vi "IsStringConstant__slk_mt.vi"(7 "create enum configure":T1, 8 "error in (no error)":errorcluster, 11 "selection list":refnum<vi>[](array[refnum])) -> (0 "error out":errorcluster, 2 "position":cluster{"Left":i32, "Top":i32}, 3 "values":string[](array[string]), 4 "not?":bool)   [LabVIEW 2010]
uses:
  TypeDef/TypeDef_CreateEnumConfigure__slk_mt.ctl
  Library/Lazyboots Menu Tool.lvlib
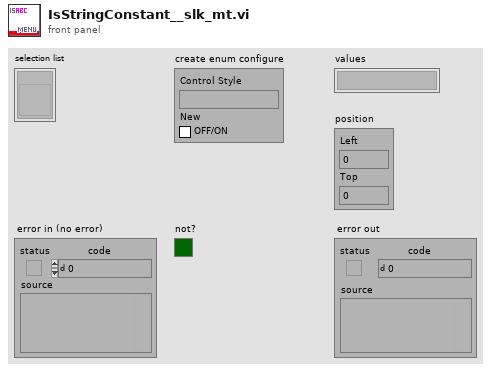
[diagram p1: front panel]
types:
  T1 = typedef "Lazyboots Menu Tool.lvlib/TypeDef_CreateEnumConfigure__slk_mt.ctl" = cluster{"Control Style":string, "New":bool}
  T2 = typedef "LVPositionTypeDef.ctl" = cluster{"Left":i32, "Top":i32}
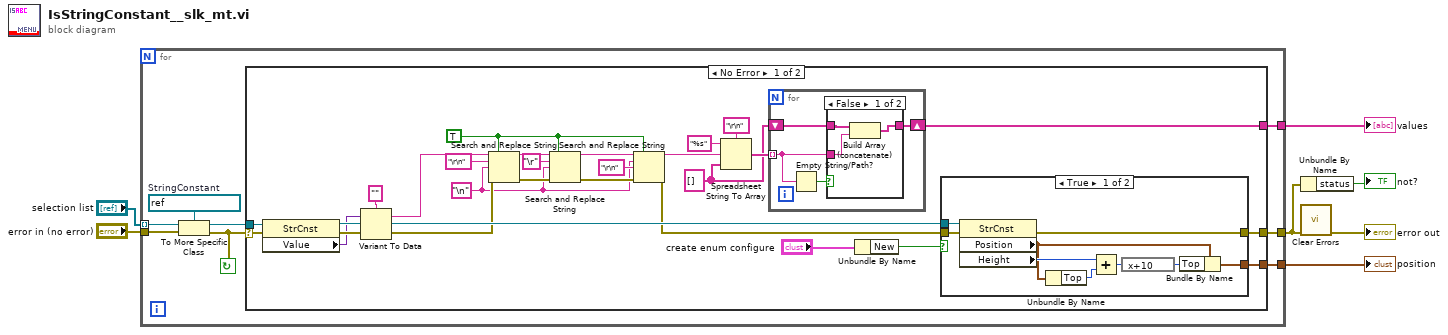
[diagram p0: block diagram]
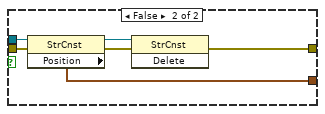
[diagram p2: hidden frame]
diagram:
  n1 = for {
    tunnel: "error in (no error)" -> [w15]
    tunnel: "selection list" -> [w13] mode=indexing
    tunnel: [w11] -> w2
    tunnel: [w9] -> w1
    tunnel: [w8] -> w3
    stop <- w12 continue-if-true
    w14 = refnum<vi> refnum  # StringConstant
    n2 = To More Specific Class(target class=w14, reference=w13, error in=w15) -> (specific class reference=w10:refnum<vi>, error out=w12:errorcluster)
    n3 = case shown="No Error" w12 {
      selector: w12 -> [w28 w67]
      tunnel: [w33 w67] -> w11
      tunnel: w10 -> [w29 _]
      tunnel: [w34 _] -> w9
      tunnel: [w27 _] -> w8
      frame No Error {
        w35 = string[] []
        w16 = "\n" ("search string")
        w17 = TRUE ("replace all? (F)")
        n4 = property class="StrCnst"(reference=w29, error in=w28) -> (reference out=w32:refnum<vi>, error out=w40:errorcluster, "Value"=w25:variant)
        n5 = Variant To Data(error in=w40, Variant=w25, type="" ("search string")) -> (error out=w26:errorcluster, data=w24:string)
        n6 = Search and Replace String(replace all?=w17, input string=w24, search string="\r\n", replace string=w16, error in=w26) -> (result string=w41:string, error out=w39:errorcluster)  [unwired: 5 out]
        n7 = Search and Replace String(replace all?=w17, input string=w41, search string="\r", replace string=w16, error in=w39) -> (result string=w21:string, error out=w19:errorcluster)  [unwired: 5 out]
        n8 = Search and Replace String(replace all?=w17, input string=w21, search string=w16, replace string="\r\n" ("replace string (\"\")"), error in=w19) -> (result string=w20:string, error out=w18:errorcluster)  [unwired: 3 in, 2 out]
        n9 = Spreadsheet String To Array(delimiter (Tab)="\r\n" ("search string"), format string="%s", spreadsheet string=w20, array type (2D Dbl)=w35) -> (array=w36:string[])
        n10 = for {
          tunnel: w36 -> [w61] mode=indexing
          shift-right: [w59] -> w34
          shift-left: w35 -> [w60]
          n11 = Empty String/Path?(string/path=w61) -> (empty?=w62:bool)
          n12 = case shown="False" w62 {
            tunnel: w61 -> [w63 _]
            tunnel: w60 -> [w65 w66]
            tunnel: [w64 w66] -> w59
            frame False {
              n13 = Build Array (concatenate)(w65, w63) -> (w64:string[])
            }
            frame True {
            }
          }
        }
        n14 = Unbundle By Name("create enum configure") -> ("New"=w30:bool)
        n15 = case shown="True" w30 {
          tunnel: w18 -> [w49 w58]
          tunnel: [w47 w53] -> w33
          tunnel: w32 -> [w48 w57]
          tunnel: [w46 w56] -> w27
          frame True {
            n16 = property class="StrCnst"(reference=w48, error in=w49) -> (error out=w47:errorcluster, "Position"=w45:T2, "Height"=w51:u32)  [unwired: 1 out]
            n17 = Unbundle By Name(w45) -> ("Top"=w50:i32)
            n18 = Add(x=w51, y=w50) -> (x+y=w52:u32)
            n19 = expression code="x+10"(w52) -> (w44:u32)
            n20 = Bundle By Name(cluster=w45, "Top"=w44) -> (w46:T2)
          }
          frame False {
            n21 = property class="StrCnst"(reference=w57, error in=w58) -> (reference out=w54:refnum<vi>, error out=w55:errorcluster, "Position"=w56:T2)
            n22 = invoke class="StrCnst" method="Delete"(reference=w54, error in=w55) -> (error out=w53:errorcluster)  [unwired: 1 in, 2 out]
          }
        }
      }
      frame Error {
      }
    }
  }
  "values" <- w1
  "position" <- w3
  n23 = Unbundle By Name(w2) -> ("status"=→"not?":bool)
  n24 = call <vilib>:"Clear Errors.vi"("error in (no error)"=w2) -> ("error out"=→"error out":errorcluster)  [unwired: 6 in]
